vi "Teleop.vi"(10 "Match Info":T3={"Autonomous Elapsed Seconds"=0.0, "TeleOp Elapsed Seconds"=0.0, "Disabled Elapsed Seconds"=0.0, "Visited Autonomous"=FALSE, "Visited TeleOp"=FALSE, "Visited Disabled"=FALSE, "Autonomous Settings"={"Autonomous Style"=enum."Independent", "VI Refnum"=refnum}}, 11 "Call Context":T4) -> ()   [LabVIEW 2016]
doc: "This VI is called for each TeleOp packet received from the DS where the robot is not disabled. It is often used to read from the joysticks and update I/O or to update setpoints for timed control loops. It should complete and return within 20 milliseconds or it may miss DS packets."
uses:
  <vilib>/Rock Robotics/WPI/DriverStation/WPI_DriverStationDerivedRobotMode.ctl
  <vilib>/Rock Robotics/WPI/DriverStation/WPI_DriverStationMatch Info.ctl
  <vilib>/Rock Robotics/WPI/ThirdParty/CanMotor/TalonSRX/WPI_CANTalonSRX_GlobalStatus.ctl
  <vilib>/Rock Robotics/WPI/ThirdParty/CanMotor/TalonSRX/WPI_CANTalonSRX_APIFeedbackSelect.ctl
  <vilib>/Rock Robotics/WPI/ThirdParty/CanMotor/TalonSRX/WPI_CANTalonSRX_APIControlMode.ctl
  <vilib>/Rock Robotics/WPI/ThirdParty/CanMotor/TalonSRX/WPI_CANTalonSRX_BrakeOverride.ctl
  <vilib>/addons/control/pid/NI_PID_pid.lvlib
  <vilib>/addons/control/pid/pid.llb/PID (DBL).vi
panel:
  out "SRX Status Right":T1
  in  "Ramp Rate":dbl format="%#_13g"
  in  "I Zone":dbl format="%#_13g"
  in  "F":dbl=0.005212 format="%#_13g"
  in  "D":dbl format="%#_13g"
  in  "I":dbl format="%#_13g"
  in  "P":dbl=0.5 format="%#_13g"
  in  "Output 3":dbl
  in  "PID gains":T2={"proportional gain (Kc)"=1.0, "integral time (Ti, min)"=0.01, "derivative time (Td, min)"=0.0} {"derivative time (Td, min)" format="%.3f"; "integral time (Ti, min)" format="%.3f"; "proportional gain (Kc)" format="%.3f"}
  in  "Range":cluster{"output high":dbl, "output low":dbl}={"output high"=100.0, "output low"=-100.0} {"output low" format="%.2f"; "output high" format="%.2f"}
  in  "Output 2":dbl format="%.2f"
  out "Output":cluster{"Sensor Velocity":dbl, dbl, dbl}(graph)
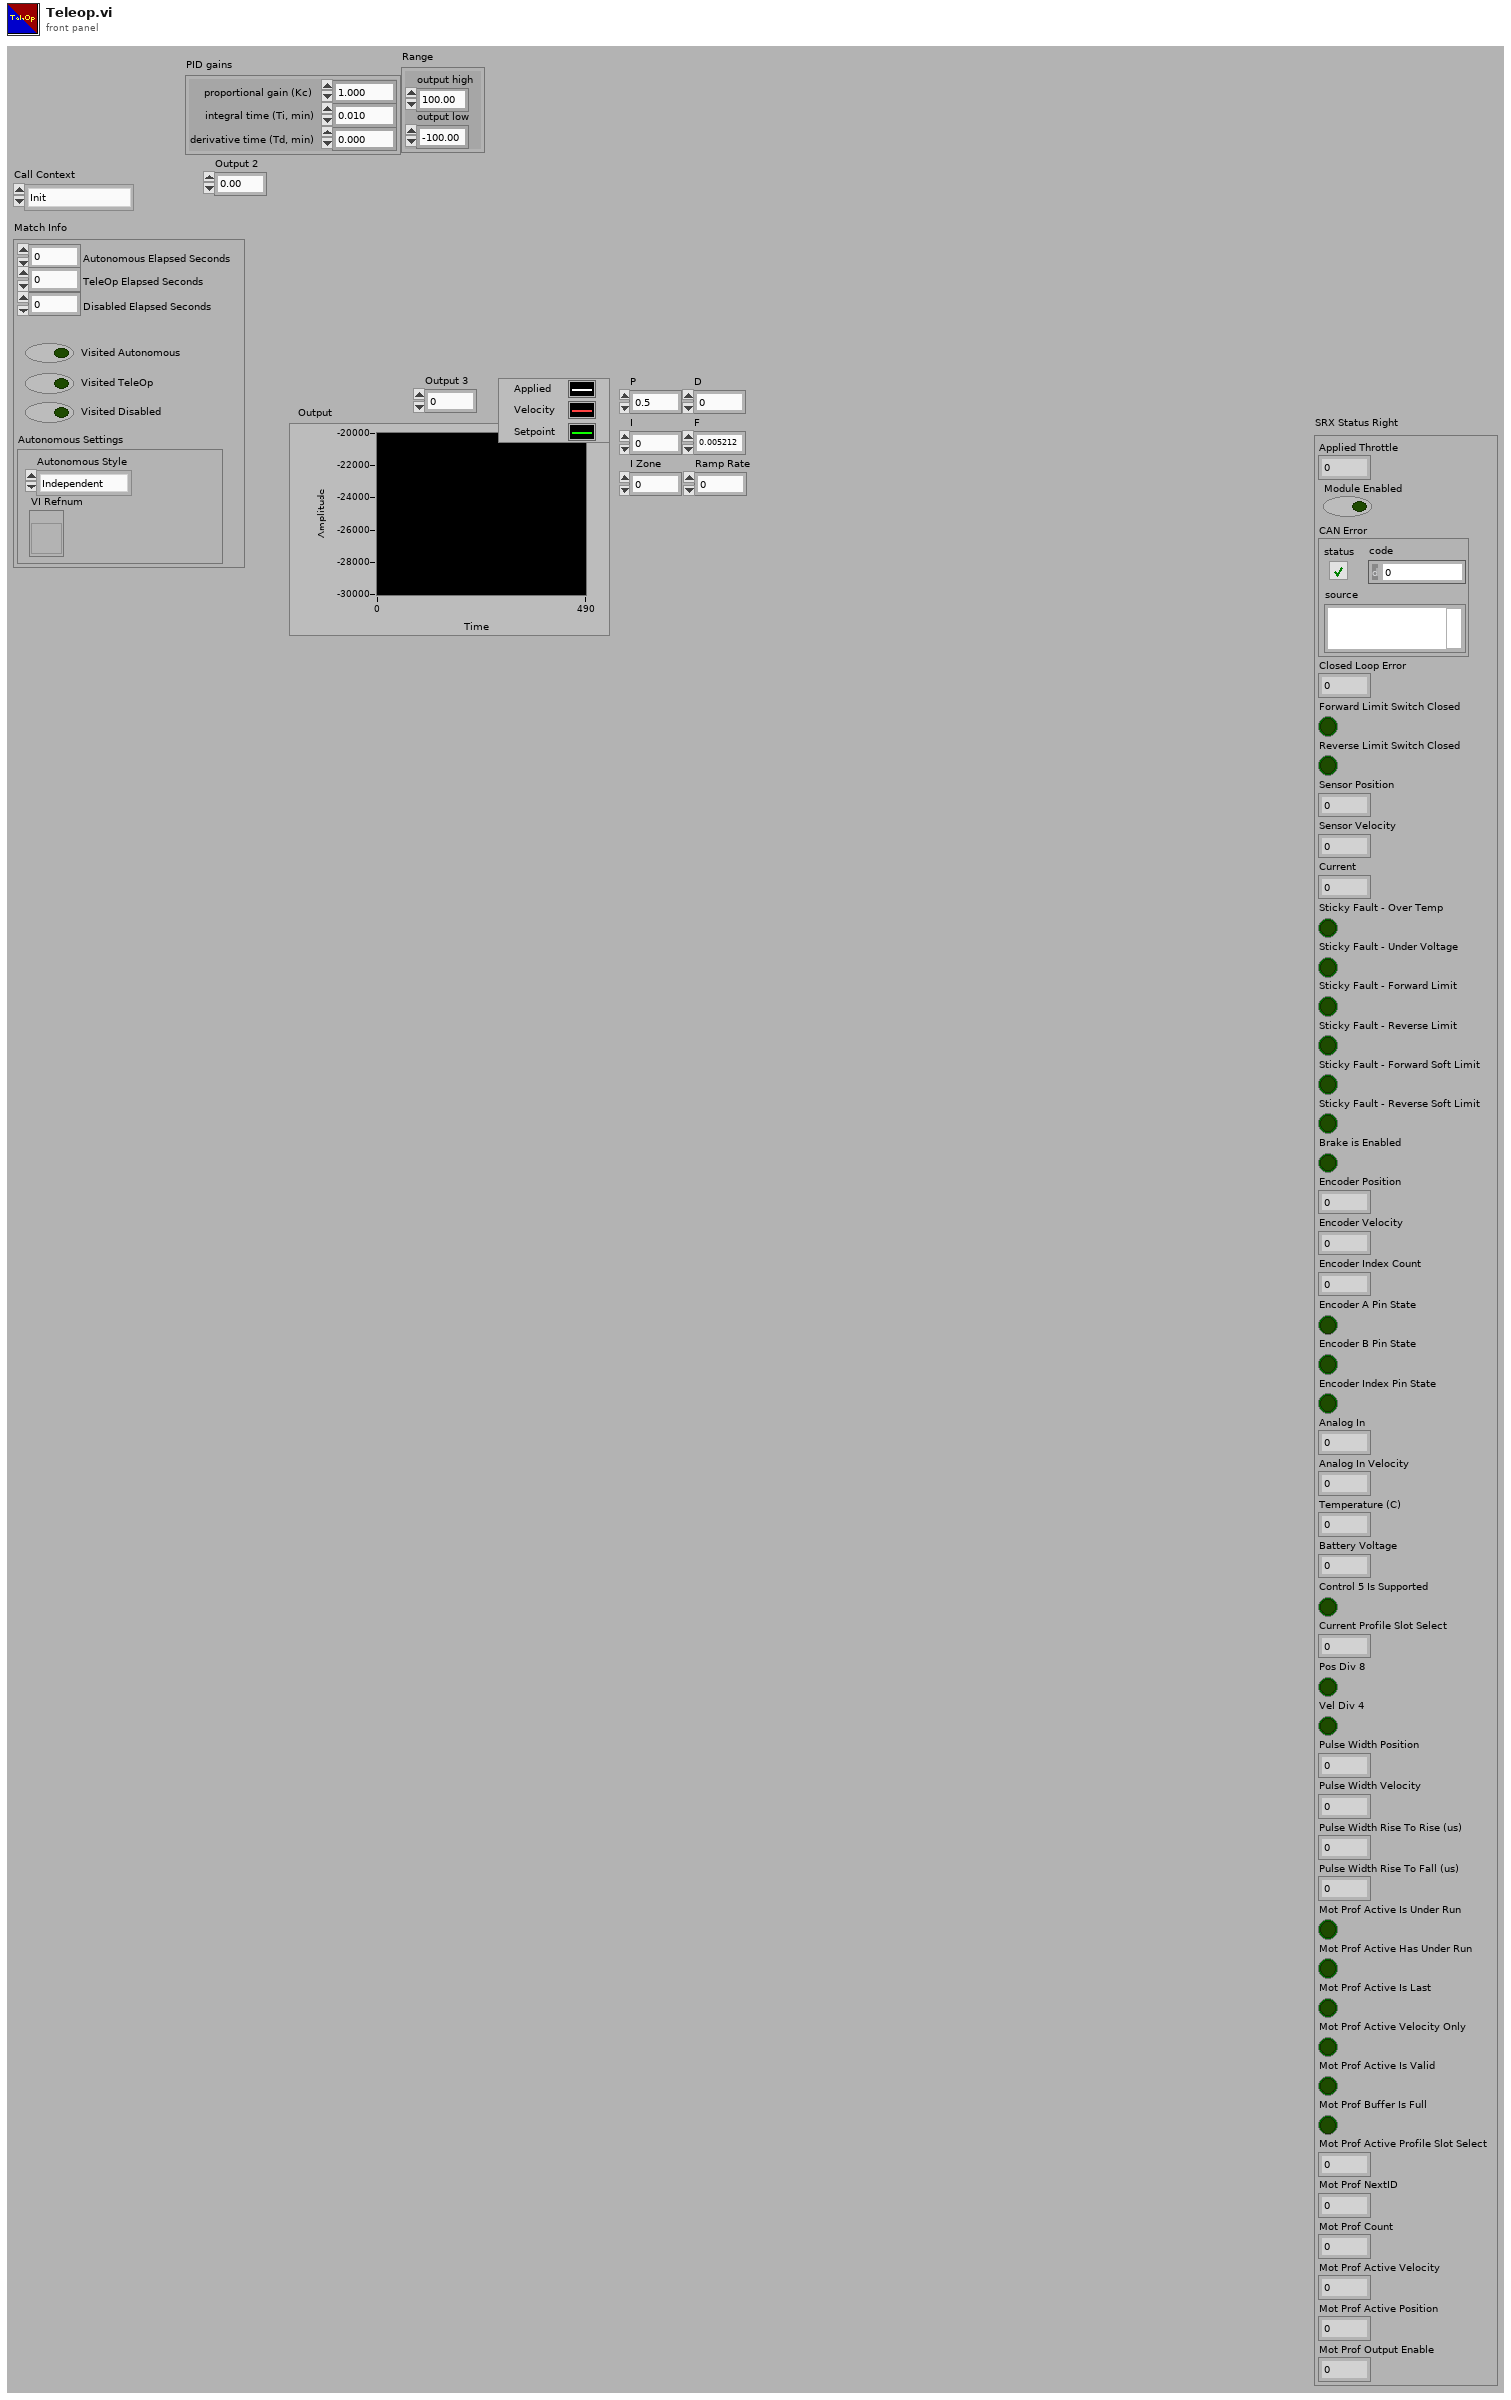
[diagram p1: front panel]
types:
  T1 = typedef "WPI_CANTalonSRX_GlobalStatus.ctl" = cluster{"Applied Throttle":dbl, "Module Enabled":bool, "CAN Error":errorcluster, "Closed Loop Error":dbl, "Forward Limit Switch Closed":bool, "Reverse Limit Switch Closed":bool, "Sensor Position":dbl, "Sensor Velocity":dbl, "Current":dbl, "Sticky Fault - Over Temp":bool, "Sticky Fault - Under Voltage":bool, "Sticky Fault - Forward Limit":bool, "Sticky Fault - Reverse Limit":bool, "Sticky Fault - Forward Soft Limit":bool, "Sticky Fault - Reverse Soft Limit":bool, "Brake is Enabled":bool, "Encoder Position":dbl, "Encoder Velocity":dbl, "Encoder Index Count":dbl, "Encoder A Pin State":bool, "Encoder B Pin State":bool, "Encoder Index Pin State":bool, "Analog In":dbl, "Analog In Velocity":dbl, "Temperature (C)":dbl, "Battery Voltage":dbl, "Control 5 Is Supported":bool, "Current Profile Slot Select":dbl, "Pos Div 8":bool, "Vel Div 4":bool, "Pulse Width Position":i32, "Pulse Width Velocity":i32, "Pulse Width Rise To Rise (us)":i32, "Pulse Width Rise To Fall (us)":i32, "Mot Prof Active Is Under Run":bool, "Mot Prof Active Has Under Run":bool, "Mot Prof Active Is Last":bool, "Mot Prof Active Velocity Only":bool, "Mot Prof Active Is Valid":bool, "Mot Prof Buffer Is Full":bool, "Mot Prof Active Profile Slot Select":i32, "Mot Prof NextID":i32, "Mot Prof Count":i32, "Mot Prof Active Velocity":dbl, "Mot Prof Active Position":dbl, "Mot Prof Output Enable":i32}
  T2 = cluster{"proportional gain (Kc)":dbl, "integral time (Ti, min)":dbl, "derivative time (Td, min)":dbl}
  T3 = typedef "WPI_DriverStationMatch Info.ctl" = cluster{"Autonomous Elapsed Seconds":dbl, "TeleOp Elapsed Seconds":dbl, "Disabled Elapsed Seconds":dbl, "Visited Autonomous":bool, "Visited TeleOp":bool, "Visited Disabled":bool, "Autonomous Settings":cluster{"Autonomous Style":enum16{"Iterative", "Independent"}, "VI Refnum":refnum<vi>}}
  T4 = typedef "WPI_DriverStationDerivedRobotMode.ctl" = enum16{"Init", "Execute", "Stop"}
  T5 = typedef "WPI_CANTalonSRX_BrakeOverride.ctl" = enum8{"No Override", "Override to Coast", "Override to Brake"}
  T6 = typedef "WPI_CANTalonSRX_APIControlMode.ctl" = enum8{"Percent VBus", "Speed", "Position", "Slave", "Unchanged / Invalid", "Voltage Compensation", "Current", "Motion Profile", "Motion Magic"}
  T7 = typedef "WPI_CANTalonSRX_APIFeedbackSelect.ctl" = enum16{"Digital Quadrature Encoder", "Analog Potentiometer", "Analog Encoder", "Count on Quad-A (Rising-Edge)", "Count on Quad-A (Falling-Edge)", "CTR Magnetic Enc (Absolute)", "CTR Magnetic Enc (Relative)", "Pulse Width"}
  T8 = typedef "WPI_MotorControlDeviceRef.ctl" = cluster{"DeviceStatus":errorcluster, "Type":T9, "PWM":cluster{"PWM Channel":T10, "DeadBand":T11}, "CAN":cluster{"Device Number":u8, "SetOutput VI Ref":variant, "GetOutput VI Ref":variant, "Enable VI Ref":variant, "Disable VI Ref":variant, "Data":variant}, "Invert":bool}
  T9 = typedef "WPI_MotorControlType.ctl" = enum16{"PWM", "CAN"}
  T10 = typedef "FPGA_DIOPWMChannel.ctl" = enum8{"PWM 0", "PWM 1", "PWM 2", "PWM 3", "PWM 4", "PWM 5", "PWM 6", "PWM 7", "PWM 8", "PWM 9", "PWM MXP 0", "PWM MXP 1", "PWM MXP 2", "PWM MXP 3", "PWM MXP 4", "PWM MXP 5", "PWM MXP 6", "PWM MXP 7", "PWM MXP 8", "PWM MXP 9", "Invalid"}
  T11 = typedef "WPI_PWMDeadband.ctl" = cluster{"Name":string, "maxPositivePwm":i32, "minPositivePwm":i32, "centerPwm":i32, "maxNegativePwm":i32, "minNegativePwm":i32, "angularRange":u16}
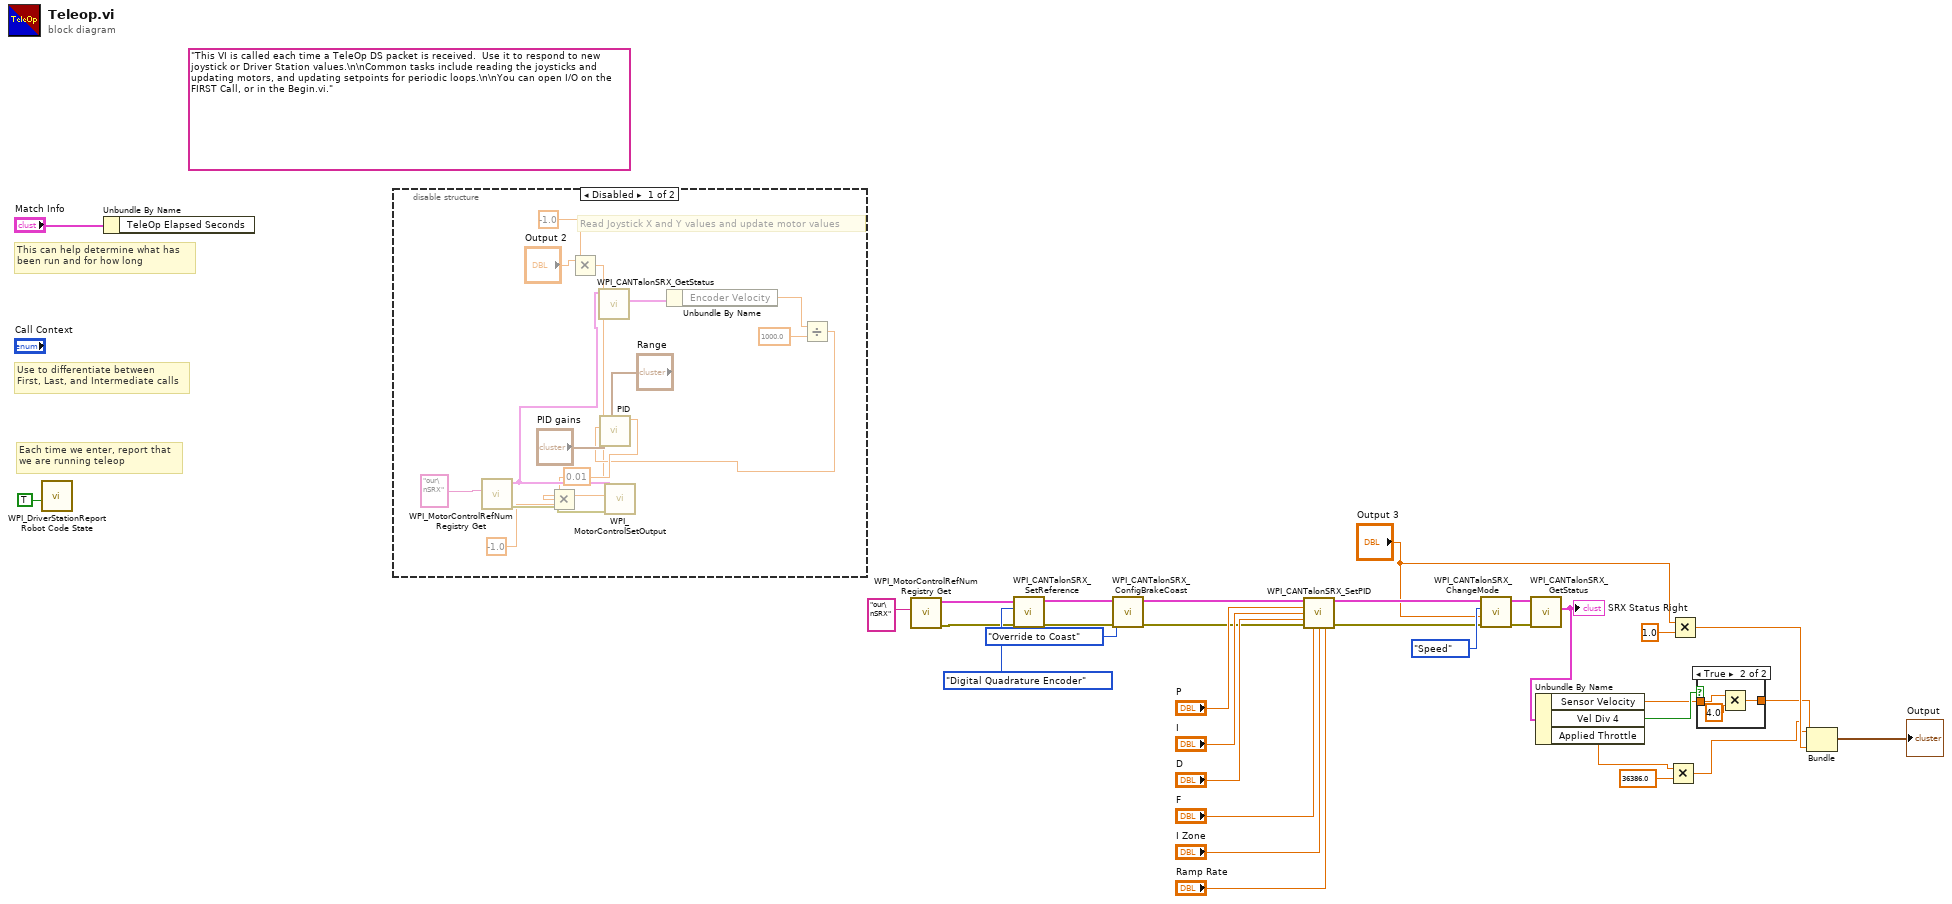
[diagram p0: block diagram]
diagram:
  (unwired) "This VI is called each time a TeleOp DS packet is received.  Use it to respond to new joystick or Driver Station values.\n\nCommon tasks include reading the joysticks and updating motors, and updating setpoints for periodic loops.\n\nYou can open I/O on the FIRST Call, or in the Begin.vi."
  # "Each time we enter, report that\nwe are running teleop"
  # "Use to differentiate between\nFirst, Last, and Intermediate calls"
  # "This can help determine what has\nbeen run and for how long"
  n1 = call <vilib>:"WPI_DriverStationReport Robot Code State.vi"("TeleOp"=TRUE ("Autonomous")) -> ()  [unwired: 10 in, 1 out]
  n2 = Unbundle By Name("Match Info") -> ()  [unwired: 1 out]
  n3 = disable-structure shown="Disabled" {
    frame Disabled {
      # "Read Joystick X and Y values and update motor values"
      n4 = call <vilib>:"WPI_MotorControlRefNum Registry Get.vi"("refnum name"="our\nSRX") -> ("error out"=w49:errorcluster, "MotorControlDevRef"=w46:T8)  [unwired: 9 in]
      n5 = Multiply(x="Output 2", y=-1.0) -> (x*y=w35:dbl)
      n6 = call <vilib>:"WPI_CANTalonSRX_GetStatus.vi"("CAN Talon SRX Ref"=w46) -> ("Talon SRX Status"=w45:T1)  [unwired: 8 in, 2 out]
      n7 = Unbundle By Name(w45) -> ("Encoder Velocity"=w39:dbl)
      n8 = Divide(x=w39, y=1000.0) -> (x/y=w38:dbl)
      n9 = call-poly <vilib>:"PID.vi"("output range"="Range", "dt (s)"=0.01, "PID gains"="PID gains", "process variable"=w38, "setpoint"=w35) -> ("output"=w43:dbl)  [unwired: 5 in, 1 out]
      n10 = Multiply(x=w43, y=-1.0) -> (x*y=w44:dbl)
      n11 = call <vilib>:"WPI_MotorControlSetOutput.vi"("error in (no error)"=w49, "Output"=w44, "MotorControlDevRef"=w46) -> ()  [unwired: 6 in, 3 out]
    }
    frame Enabled {
    }
  }
  n12 = call <vilib>:"WPI_MotorControlRefNum Registry Get.vi"("refnum name"="our\nSRX") -> ("error out"=w12:errorcluster, "MotorControlDevRef"=w13:T8)  [unwired: 9 in]
  n13 = call <vilib>:"WPI_CANTalonSRX_SetReference.vi"("error in (no error)"=w12, "Feedback Reference"=WPI_CANTalonSRX_APIFeedbackSelect."Digital Quadrature Encoder", "CAN Talon SRX Ref"=w13) -> ("error out"=w19:errorcluster, "CAN Talon SRX Ref"=w20:T8)  [unwired: 7 in]
  n14 = call <vilib>:"WPI_CANTalonSRX_ConfigBrakeCoast.vi"("error in (no error)"=w19, "Brake / Coast Mode"=WPI_CANTalonSRX_BrakeOverride."Override to Coast", "CAN Talon SRX Ref"=w20) -> ("error out"=w17:errorcluster, "CAN Talon SRX Ref"=w18:T8)  [unwired: 7 in]
  n15 = call <vilib>:"WPI_CANTalonSRX_SetPID.vi"("CAN Talon SRX Ref"=w18, "P"="P", "I"="I", "D"="D", "error in (no error)"=w17, "F"="F", "I Zone"="I Zone", "Ramp Rate"="Ramp Rate") -> ("CAN Talon SRX Ref"=w22:T8, "error out"=w21:errorcluster)  [unwired: 6 in]
  n16 = call <vilib>:"WPI_CANTalonSRX_ChangeMode.vi"("error in (no error)"=w21, "Output"="Output 3", "Control Mode"=WPI_CANTalonSRX_APIControlMode."Speed", "CAN Talon SRX Ref"=w22) -> ("error out"=w16:errorcluster, "CAN Talon SRX Ref"=w15:T8)  [unwired: 6 in]
  n17 = call <vilib>:"WPI_CANTalonSRX_GetStatus.vi"("error in (no error)"=w16, "CAN Talon SRX Ref"=w15) -> ("Talon SRX Status"=w14:T1)  [unwired: 7 in, 2 out]
  "SRX Status Right" <- w14
  n18 = Unbundle By Name(w14) -> ("Sensor Velocity"=w9:dbl, "Vel Div 4"=w10:bool, "Applied Throttle"=w6:dbl)
  n19 = Multiply(x=w6, y=36386.0) -> (x*y=w2:dbl)
  n20 = Multiply(x="Output 3", y=1.0) -> (x*y=w3:dbl)
  n21 = case shown="True" w10 {
    tunnel: w9 -> [w50 w52]
    tunnel: [w50 w53] -> w1
    frame False {
    }
    frame True {
      n22 = Multiply(x=w52, y=4.0) -> (x*y=w53:dbl)
    }
  }
  n23 = Bundle(w2, "Sensor Velocity"=w1, w3) -> (→"Output":cluster{dbl, "Sensor Velocity":dbl, dbl})  [unwired: 1 in]
